vi "DrawLevels.vi"(8 "SAC/FAC":bool=TRUE, 10 "Size":i32, 11 "Ind":i32) -> (3 "Array":cluster{"theta (deg)":i32, i32}[](array[cluster]))   [LabVIEW 2017]
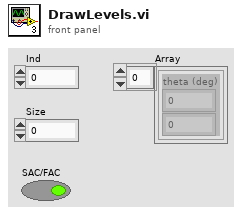
[diagram p1: front panel]
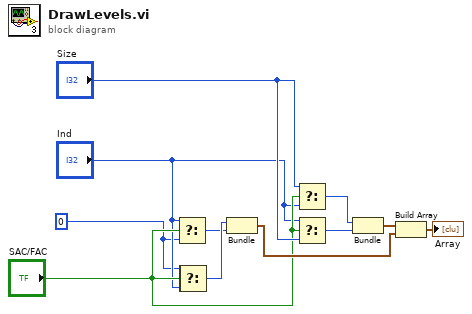
[diagram p0: block diagram]
diagram:
  w1 = 0 ("theta (deg)")
  n1 = Select(t="Ind", s="SAC/FAC", f=w1) -> (s? t:f=w7:i32)
  n2 = Select(t=w1, s="SAC/FAC", f="Ind") -> ()  [unwired: 1 out]
  n3 = Select(t=w1, s="SAC/FAC", f="Ind") -> (s? t:f=w8:i32)
  n4 = Bundle("Ind"=w8, "theta (deg)"=w7) -> (w10:cluster{"Ind":i32, "theta (deg)":i32})  [unwired: 1 in]
  n5 = Select(t="Size", s="SAC/FAC", f="Ind") -> (s? t:f=w5:i32)
  n6 = Select(t="Ind", s="SAC/FAC", f="Size") -> (s? t:f=w6:i32)
  n7 = Bundle("Ind"=w5, "Size"=w6) -> (w9:cluster{"Ind":i32, "Size":i32})  [unwired: 1 in]
  n8 = Build Array(w9, w10) -> (→"Array":cluster{"Ind":i32, "theta (deg)":i32}[])
